vi "Check if MES Failed.vi"(11 "Results of the roccesses":string[](array[string])) -> (2 "Connection error":bool, 3 "MES Failed":bool)   [LabVIEW 2025, in "MES Interlcok.lvlib"]
uses:
  MES Interlcok.lvlib
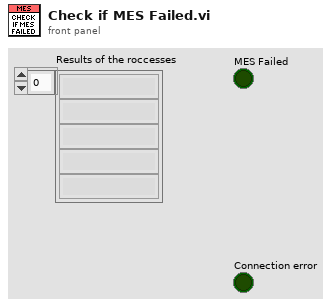
[diagram p1: front panel]
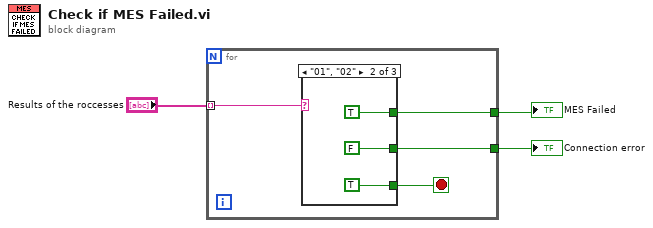
[diagram p0: block diagram]
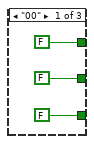
[diagram p2: hidden frame]
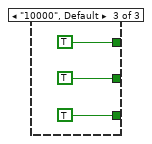
[diagram p3: hidden frame]
diagram:
  n1 = for {
    tunnel: "Results of the roccesses" -> [w7] mode=indexing
    tunnel: [w5] -> w2
    tunnel: [w4] -> w1
    stop <- w6 stop-if-true
    n2 = case shown="\"01\", \"02\"" w7 {
      tunnel: [FALSE TRUE TRUE] -> w6
      tunnel: [FALSE ("MES Failed") TRUE ("MES Failed") TRUE ("MES Failed")] -> w5
      tunnel: [FALSE ("Connection error") FALSE ("Connection error") TRUE ("Connection error")] -> w4
      frame "00" {
      }
      frame "01", "02" {
      }
      frame "10000", Default {
      }
    }
  }
  "MES Failed" <- w2
  "Connection error" <- w1
